vi "set_config_cluster.vi"(8 "error in (no error)":errorcluster, 10 "config cluster variant":variant, 11 "DetectorYK090623DAQmxAnalog in":refnum<class "DetectorYK090623DAQmxAnalog.lvclass">) -> (0 "error out":errorcluster, 3 "DetectorYK090623DAQmxAnalog out":refnum<class "DetectorYK090623DAQmxAnalog.lvclass">)   [LabVIEW 2010, in "DetectorYK090623DAQmxAnalog.lvclass"]
uses:
  DetectorYK090623DAQmxAnalog.lvclass
  DetectorYK090623DAQmxAnalog.lvclass/DetectorYK090623DAQmxAnalog.ctl
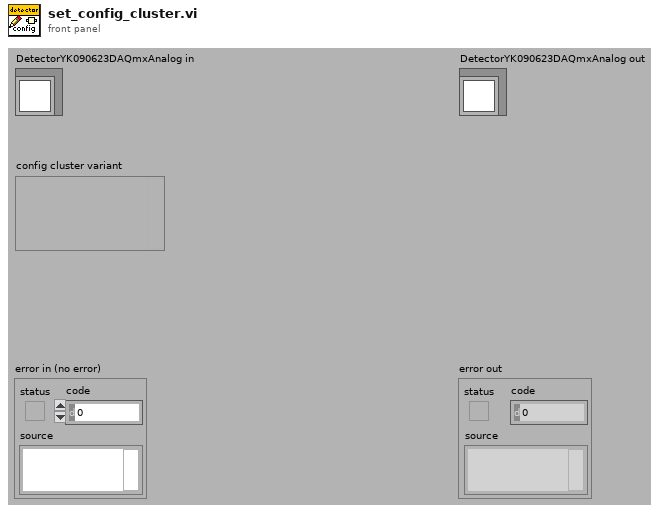
[diagram p1: front panel]
types:
  T1 = typedef "DetectorYK090623DAQmxAnalog.lvclass/config_data_cluster.ctl" = cluster{"default voltage":dbl[unit], "analog out":T2}
  T2 = typedef "plugin_specification.ctl" = cluster{"class path":string, "configuration":string, "label":string, "settings name":string}
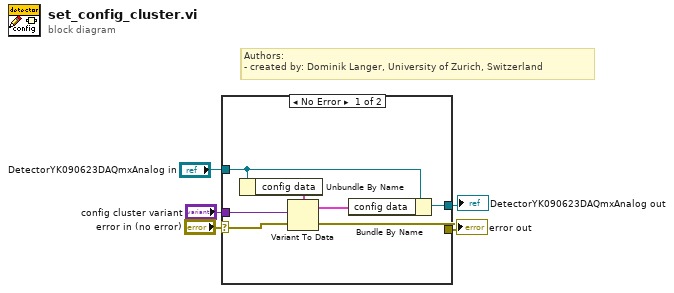
[diagram p0: block diagram]
diagram:
  # "Authors: \n- created by: Dominik Langer, University of Zurich, Switzerland"
  # "Authors: \n- created by: Dominik Langer, University of Zurich, Switzerland"
  n1 = case shown="No Error" "error in (no error)" {
    selector: "error in (no error)" -> [w9 w13]
    tunnel: "DetectorYK090623DAQmxAnalog in" -> [w8 w14]
    tunnel: [w6 w14] -> w2
    tunnel: [w7 w13] -> w1
    tunnel: "config cluster variant" -> [w10 _]
    frame No Error {
      n2 = Unbundle By Name(w8) -> ("config data"=w11:T1)
      n3 = Variant To Data(error in=w9, Variant=w10, type=w11) -> (error out=w7:errorcluster, data=w12:T1)
      n4 = Bundle By Name(cluster=w8, "config data"=w12) -> (w6:refnum<class "DetectorYK090623DAQmxAnalog.lvclass">)
    }
    frame Error {
    }
  }
  "error out" <- w1
  "DetectorYK090623DAQmxAnalog out" <- w2
